vi "Communication Worker.vi"(8 "error in (no error)":errorcluster, 11 "IP Connection in":refnum<class "IP Connection.lvclass">) -> (0 "error out":errorcluster, 3 "IP Connection out":refnum<class "IP Connection.lvclass">)   [LabVIEW 2011, in "Tinkerforge.lvlib" / "IP Connection.lvclass"]
doc: "This VI handles the complete TCP/IP communication of this IP Connection object."
uses:
  IP Connection.lvclass
  IP Connection.lvclass/IP Connection.ctl
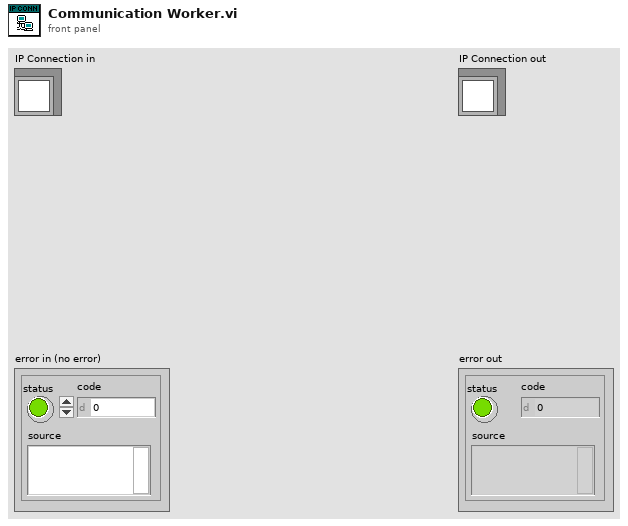
[diagram p1: front panel]
types:
  T1 = typedef "Tinkerforge.lvlib/IP Connection.lvclass/Message.ctl" = cluster{"Stack ID":u8, "Function ID":u8, "Data":string, "Request GUID":string, "Timeout":i32, "Response":bool}
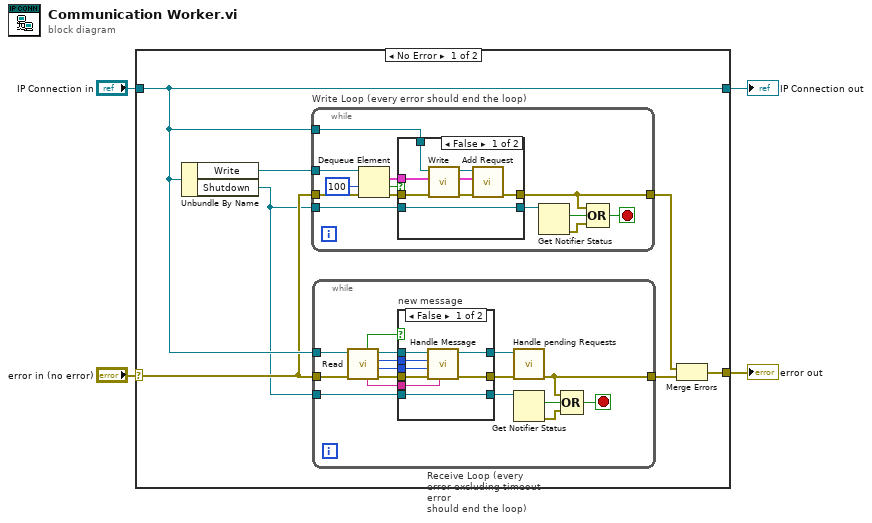
[diagram p0: block diagram]
diagram:
  n1 = case shown="No Error" "error in (no error)" {
    selector: "error in (no error)" -> [w8 w61]
    tunnel: [w10 w61] -> w3
    tunnel: [w9 w60] -> w1
    tunnel: "IP Connection in" -> [w9 w60]
    frame No Error {
      n2 = Unbundle By Name(w9) -> ("Write"=w11:refnum<queue>, "Shutdown"=w5:refnum<notifier>)
      n3 = while "Write Loop (every error should end the loop)" {
        tunnel: w8 -> [w50]
        tunnel: w11 -> [w49]
        tunnel: w9 -> [w47]
        tunnel: [w38] -> w7
        tunnel: w5 -> [w42]
        stop <- w39 stop-if-true
        n4 = Dequeue Element(queue=w49, timeout in ms (-1)=100, error in (no error)=w50) -> (element=w46:T1, timed out?=w43:bool, error out=w48:errorcluster)  [unwired: 1 out]
        n5 = case shown="False" w43 {
          tunnel: w48 -> [w57 w58]
          tunnel: w47 -> [w56 _]
          tunnel: w46 -> [w55 _]
          tunnel: [w52 w58] -> w38
          tunnel: w42 -> [w51 w59]
          tunnel: [w51 w59] -> w41
          frame False {
            n6 = call "Write.vi"("error in (no error)"=w57, "Write Data"=w55, "IP Connection in"=w56) -> ("error out"=w54:errorcluster, "IP Connection out"=w53:refnum<class "IP Connection.lvclass">)  [unwired: 7 in]
            n7 = call "Add Request.vi"("error in (no error)"=w54, "Write Data"=w55, "IP Connection in"=w53) -> ("error out"=w52:errorcluster)  [unwired: 7 in, 1 out]
          }
          frame True {
          }
        }
        n8 = Get Notifier Status(notifier=w41) -> (current notification=w45:bool, error out=w44:errorcluster)  [unwired: 1 in, 3 out]
        n9 = Compound Arithmetic op=OR(w38, w45, w44) -> (w39:bool)
      }
      n10 = while "Receive Loop (every error excluding timeout error\nshould end the loop)" {
        tunnel: w8 -> [w27]
        tunnel: w9 -> [w26]
        tunnel: [w14] -> w6
        tunnel: w5 -> [w13]
        stop <- w15 stop-if-true
        n11 = call "Read.vi"("error in (no error)"=w27, "IP Connection in"=w26) -> ("error out"=w25:errorcluster, "Function ID"=w22:u8, "Stack ID"=w23:u8, "IP Connection out"=w24:refnum<class "IP Connection.lvclass">, "Data"=w21:string, "timed out"=w20:bool)  [unwired: 4 in]
        n12 = case "new message" shown="False" w20 {
          tunnel: w25 -> [w35 _]
          tunnel: [w34 _] -> w18
          tunnel: w24 -> [w33 w37]
          tunnel: w23 -> [w32 _]
          tunnel: w22 -> [w31 _]
          tunnel: w21 -> [w30 _]
          tunnel: [w29 w37] -> w19
          tunnel: w13 -> [w28 w36]
          tunnel: [w28 w36] -> w12
          frame False {
            n13 = call "Handle Message.vi"("Data"=w30, "error in (no error)"=w35, "Function ID"=w31, "Stack ID"=w32, "IP Connection in"=w33) -> ("error out"=w34:errorcluster, "IP Connection out"=w29:refnum<class "IP Connection.lvclass">)  [unwired: 5 in]
          }
          frame True {
            # "clear\ntimeout\nerror"
          }
        }
        n14 = call "Handle pending Requests.vi"("error in (no error)"=w18, "IP Connection in"=w19) -> ("error out"=w14:errorcluster)  [unwired: 8 in, 1 out]
        n15 = Get Notifier Status(notifier=w12) -> (current notification=w17:bool, error out=w16:errorcluster)  [unwired: 1 in, 3 out]
        n16 = Compound Arithmetic op=OR(w14, w17, w16) -> (w15:bool)
      }
      n17 = Merge Errors(w7, w6) -> (w10:errorcluster)
    }
    frame Error {
    }
  }
  "error out" <- w3
  "IP Connection out" <- w1
